vi "outputs.vi"() -> ()   [LabVIEW 2019]
panel:
  out "Talon 2 Speed":dbl
  out "Talon 1 Speed":dbl
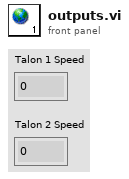
[diagram p1: front panel]
diagram:
